vi "logMsg.vi"(8 "error in (no error)":errorcluster, 9 "msg":string, 10 "type":T1(ring), 11 "Logger in":refnum<class "Logger.lvclass">) -> (0 "error out":errorcluster, 2 "msgLog":string, 3 "Logger out":refnum<class "Logger.lvclass">)   [LabVIEW 2018, in "Logger.lvclass"]
doc: "Log the message. This function will check the counter of record, and decide to create the new log file or not."
uses:
  Logger.lvclass
  Logger.lvclass/Logger.ctl
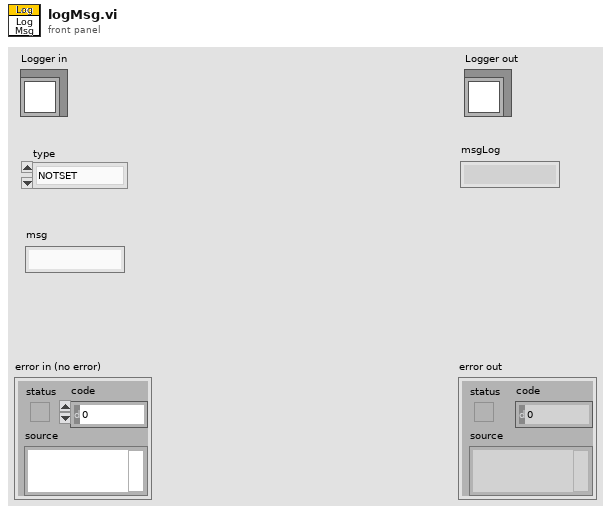
[diagram p1: front panel]
types:
  T1 = enum16{"NOTSET", "DEBUG", "INFO", "WARNING", "ERROR", "CRITICAL"}
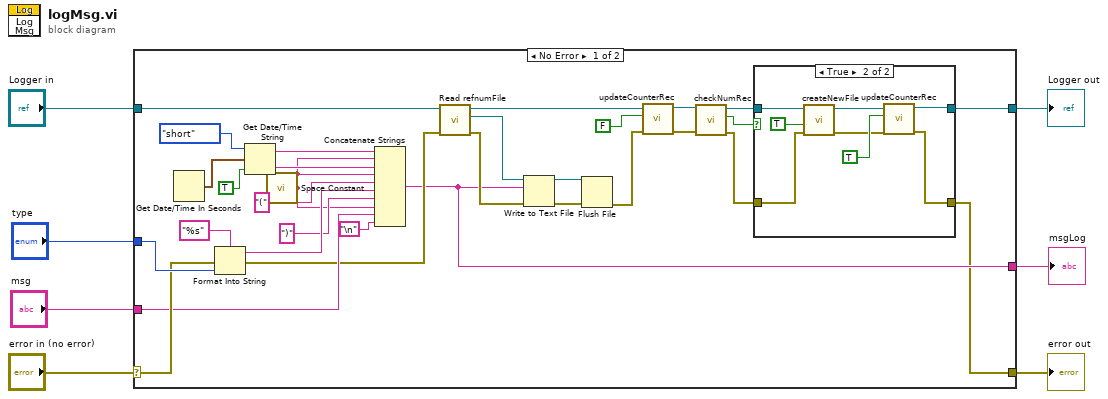
[diagram p0: block diagram]
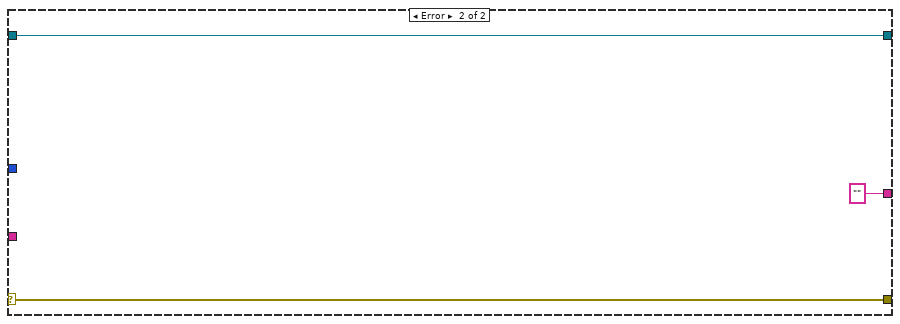
[diagram p3: hidden frame]
diagram:
  n1 = case shown="No Error" "error in (no error)" {
    selector: "error in (no error)" -> [w32 w51]
    tunnel: [w8 w51] -> w6
    tunnel: [w9 w50] -> w4
    tunnel: "Logger in" -> [w24 w50]
    tunnel: "type" -> [w33 _]
    tunnel: "msg" -> [w26 _]
    tunnel: [w15 ""] -> w1
    frame No Error {
      n2 = Get Date/Time In Seconds() -> (seconds since 1Jan1904=w38:timestamp)
      n3 = Format Into String(format string="%s", error in=w32, w33) -> (resulting string=w29:string, error out=w23:errorcluster)  [unwired: 1 in]
      n4 = Get Date/Time String(date format (0)=enum16{"short", "long", "abbreviated"}."short", seconds (now)=w38, want seconds? (F)=TRUE) -> (date string=w35:string, time string=w34:string)
      n5 = call <vilib>:"Space Constant.vi"() -> ("String"=w27:string)
      n6 = Concatenate Strings(w35, w27, w34, w27, "(", w29, ")", w27, w26, "\n") -> (w15:string)
      n7 = call "Read refnumFile.vi"("error in (no error)"=w23, "Logger in"=w24) -> ("error out"=w21:errorcluster, "refnumFile"=w22:refnum<file>, "Logger out"=w18:refnum<class "Logger.lvclass">)  [unwired: 7 in]
      n8 = Write to Text File(file (use dialog)=w22, text=w15, error in=w21) -> (refnum out=w20:refnum<file>, error out=w19:errorcluster)  [unwired: 1 in, 1 out]
      n9 = Flush File(refnum=w20, error in=w19) -> (error out=w16:errorcluster)  [unwired: 1 out]
      n10 = call "updateCounterRec.vi"("error in (no error)"=w16, "reset"=FALSE, "Logger in"=w18) -> ("error out"=w13:errorcluster, "Logger out"=w14:refnum<class "Logger.lvclass">)  [unwired: 7 in]
      n11 = call "checkNumRec.vi"("error in (no error)"=w13, "Logger in"=w14) -> ("error out"=w10:errorcluster, "isToCreateNewFile"=w12:bool, "Logger out"=w11:refnum<class "Logger.lvclass">)  [unwired: 7 in]
      n12 = case shown="True" w12 {
        tunnel: w11 -> [w40 w48]
        tunnel: w10 -> [w39 w46]
        tunnel: [w40 w41] -> w9
        tunnel: [w39 w42] -> w8
        frame False {
        }
        frame True {
          n13 = call "createNewFile.vi"("error in (no error)"=w46, "isNewFilePathFromCounter"=TRUE, "Logger in"=w48) -> ("error out"=w43:errorcluster, "Logger out"=w45:refnum<class "Logger.lvclass">)  [unwired: 7 in]
          n14 = call "updateCounterRec.vi"("error in (no error)"=w43, "reset"=TRUE, "Logger in"=w45) -> ("error out"=w42:errorcluster, "Logger out"=w41:refnum<class "Logger.lvclass">)  [unwired: 7 in]
        }
      }
    }
    frame Error {
    }
  }
  "error out" <- w6
  "Logger out" <- w4
  "msgLog" <- w1
